vi "Ping Test Executer.vi"(8 "Error in (no error)":errorcluster) -> (0 "Error Out":errorcluster, 3 "% packets returned":dbl)   [LabVIEW 2017]
panel:
  out "String":string
  in  "IP Address":string
  in  "timeout(ms)":i32
  in  "Ping Count":i32
  in  "Packet Size":i32
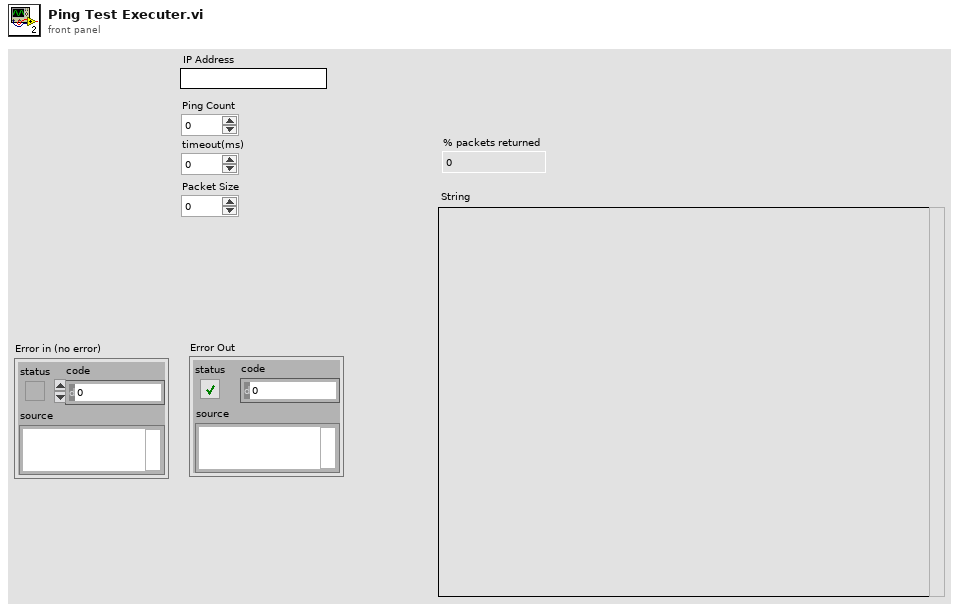
[diagram p1: front panel]
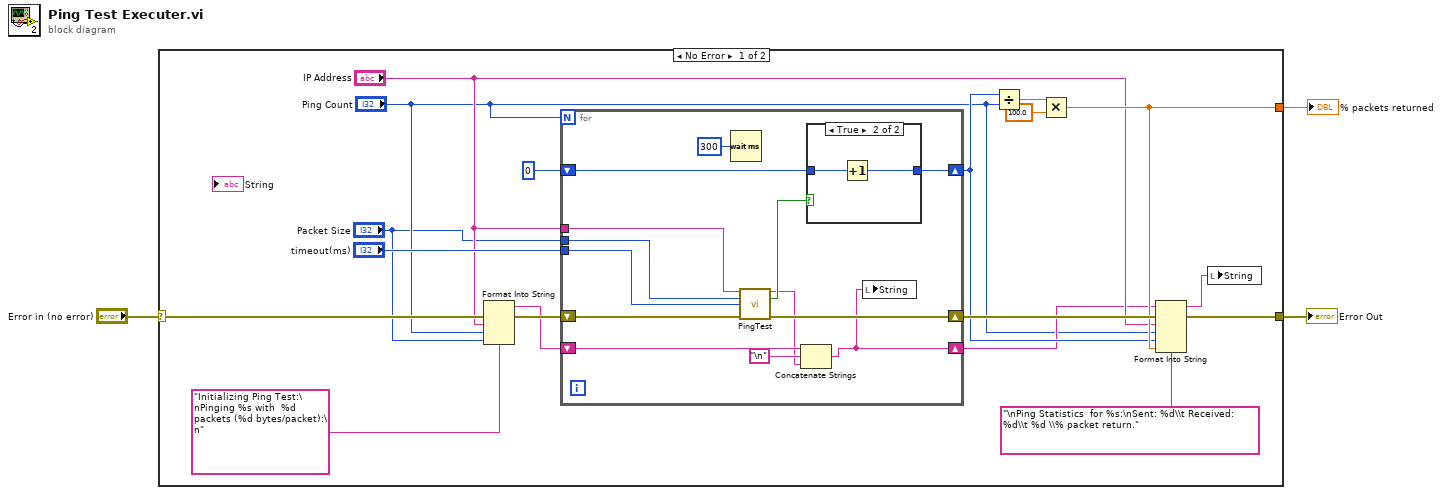
[diagram p0: block diagram]
diagram:
  n1 = case shown="No Error" "Error in (no error)" {
    selector: "Error in (no error)" -> [w21 w38]
    tunnel: [w12 w38] -> w2
    tunnel: [w9 _] -> w1
    frame No Error {
      n2 = Format Into String(format string="Initializing Ping Test:\nPinging %s with  %d packets (%d bytes/packet):\n", error in=w21, "IP Address", "Ping Count", "Packet Size") -> (resulting string=w14:string, error out=w20:errorcluster)  [unwired: 1 in]
      n3 = for {
        N: "Ping Count" -> [_]
        tunnel: "IP Address" -> [w34]
        tunnel: "Packet Size" -> [w33]
        tunnel: "timeout(ms)" -> [w32]
        shift-right: [w30] -> w13
        shift-left: w20 -> [w31]
        shift-right: [w27] -> w8
        shift-left: 0 -> [w28]
        shift-right: [w25] -> w6
        shift-left: w14 -> [w26]
        n4 = Wait (ms)(milliseconds to wait=u32 300) -> ()  [unwired: 1 out]
        n5 = call "PingTest.vi"("IP/Address"=w34, "PacketSize"=w33, "timeout"=w32, "Error in (no error)"=w31) -> ("Response"=w23:string, "PingSuccess?"=w29:bool, "Error out"=w30:errorcluster)  [unwired: 9 in]
        n6 = Concatenate Strings(w26, "\n", w23) -> (w25:string)
        n7 = case shown="True" w29 {
          tunnel: w28 -> [w35 w37]
          tunnel: [w35 w36] -> w27
          frame False {
          }
          frame True {
            n8 = Increment(x=w37) -> (x+1=w36:i32)
          }
        }
        n9 = local write "String"(w25) -> ()
      }
      n10 = Divide(x=w8, y="Ping Count") -> (x/y=w16:dbl)
      n11 = Multiply(x=w16, y=100.0) -> (x*y=w9:dbl)
      n12 = Format Into String(format string="\nPing Statistics  for %s:\nSent: %d\\t Received: %d\\t %d \\% packet return.", initial string=w6, error in=w13, "IP Address", "Ping Count", w8, w9) -> (resulting string=w10:string, error out=w12:errorcluster)
      n13 = local write "String"(w10) -> ()
    }
    frame Error {
    }
  }
  "Error Out" <- w2
  "% packets returned" <- w1
